vi "Init Save Image Class.vi"(8 "error in (no error)":errorcluster, 11 "Simulated_Image_Constructor in":refnum<class "Simulated_Image_Constructor.lvclass">) -> (0 "error out":errorcluster, 3 "Simulated_Image_Constructor out":refnum<class "Simulated_Image_Constructor.lvclass">)   [LabVIEW 2018, in "Simulated_Image_Constructor.lvclass"]
uses:
  Simulated_Image_Constructor.lvclass
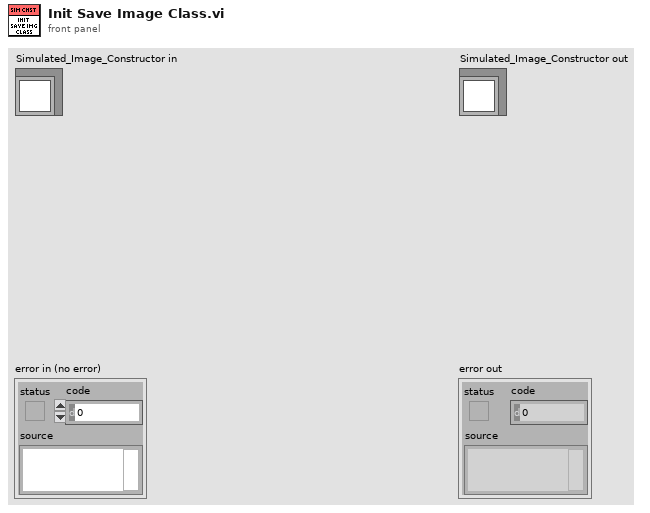
[diagram p1: front panel]
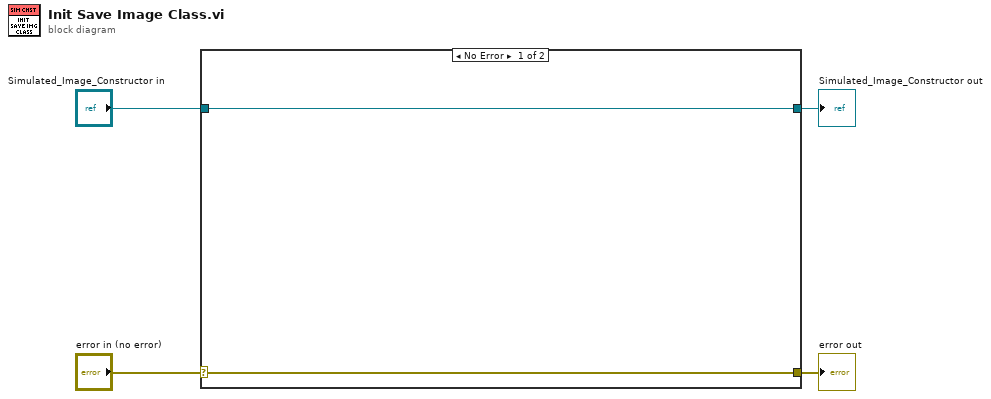
[diagram p0: block diagram]
diagram:
  n1 = case shown="No Error" "error in (no error)" {
    selector: "error in (no error)" -> [w5 w8]
    tunnel: [w5 w8] -> w3
    tunnel: [w6 w7] -> w1
    tunnel: "Simulated_Image_Constructor in" -> [w6 w7]
    frame No Error {
    }
    frame Error {
    }
  }
  "error out" <- w3
  "Simulated_Image_Constructor out" <- w1
